vi "MoveSnakes.vi"(8 "error in (no error)":errorcluster, 10 "Engine in":refnum<class "Engine.lvclass">, 11 "PongDemo in":refnum<class "PongDemo.lvclass">) -> (0 "error out":errorcluster, 2 "Engine out":refnum<class "Engine.lvclass">, 3 "PongDemo out":refnum<class "PongDemo.lvclass">)   [LabVIEW 2019, in "RT_Game.lvlib" / "PongDemo.lvclass"]
uses:
  PongDemo.lvclass
  C:/Users/FreshBob/Dropbox/VIs/myRIO_GameConsole/RT/RT_Game/Pong/Pong.lvclass
  Engine/Engine.lvclass
  Pong/Pong.lvclass/Pong.ctl
  Pong/Read left_panel.vi
  Pong/Read ball.vi
  Pong/Read right_panel.vi
  Pong/Read pause_time.vi
  Pong/Write left_panel.vi
  Pong/Write right_panel.vi
  PongPanel/PongPanel.lvclass
  PongBall/PongBall.lvclass
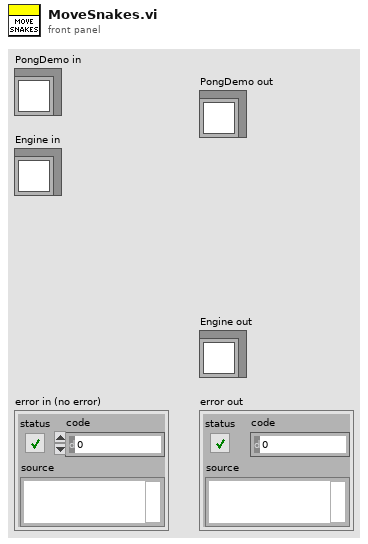
[diagram p1: front panel]
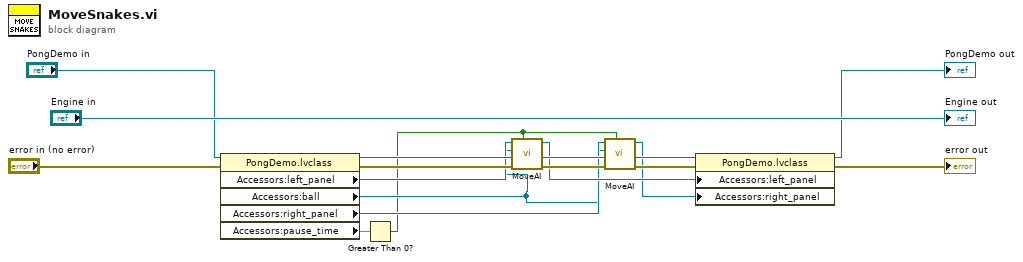
[diagram p0: block diagram]
diagram:
  n1 = property class="PongDemo.lvclass"(reference="PongDemo in", error in="error in (no error)") -> (reference out=w11:refnum<class "PongDemo.lvclass">, error out=w14:errorcluster, "Accessors:left_panel"=w8:refnum<class "PongPanel.lvclass">, "Accessors:ball"=w3:refnum<class "PongBall.lvclass">, "Accessors:right_panel"=w5:refnum<class "PongPanel.lvclass">, "Accessors:pause_time"=w2:dbl)
  n2 = Greater Than 0?(x=w2) -> (x > 0?=w1:bool)
  n3 = call "MoveAI.vi"("ReturnHome(F)"=w1, "error in (no error)"=w14, "Ball"=w3, "PongPanel in"=w8) -> ("error out"=w9:errorcluster, "PongPanel out"=w7:refnum<class "PongPanel.lvclass">)  [unwired: 6 in]
  n4 = call "MoveAI.vi"("ReturnHome(F)"=w1, "error in (no error)"=w9, "Ball"=w3, "PongPanel in"=w5) -> ("error out"=w6:errorcluster, "PongPanel out"=w4:refnum<class "PongPanel.lvclass">)  [unwired: 6 in]
  n5 = property class="PongDemo.lvclass"(reference=w11, error in=w6, "Accessors:left_panel"=w7, "Accessors:right_panel"=w4) -> (reference out=→"PongDemo out":refnum<class "PongDemo.lvclass">, error out=→"error out":errorcluster)
  "Engine out" <- "Engine in"
